vi "Initialize_Flatten.vi"(8 "error in":errorcluster, 10 "InstanceName":string, 11 "ChillerNew.lvclass":refnum<class "ChillerNew.lvclass">) -> (0 "error out":errorcluster, 3 "output cluster":refnum<class "ChillerNew.lvclass">)   [LabVIEW 2023, in "ChillerNew.lvclass"]
uses:
  ChillerNew.lvclass
  ChillerNew.lvclass/ChillerNew.ctl
  287c8f4c-a7e3-4bef-a246-9f8e491f331f.vi
  026c2e1f-36c0-42b1-b36e-75aff64539ee.vi
  f03e60db-0e78-4351-a110-c32dc1ba0a1a.vi
  838db0e1-c7d3-41be-87a2-4c748dcee471.vi
  026c2e1f-36c0-42b1-b36e-75aff64539ee.vi/4bc1c15b-36ab-481f-b8dd-c64075ce723a.vi
  838db0e1-c7d3-41be-87a2-4c748dcee471.vi/4bc1c15b-36ab-481f-b8dd-c64075ce723a.vi
  <vilib>/ADAS Replay HIL/AdasHilServices/AdasHilServices Fill In Error Info Ex.vi
  <vilib>/Utility/Data Type/NI_Data Type.lvlib
  AdasHilServices.dll
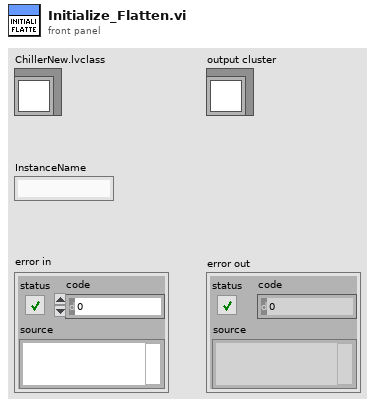
[diagram p1: front panel]
types:
  T1 = cluster{"OnOffCtl":bool, "SP1":dbl, "Watchdog":i32}
  T2 = cluster{"OnOffSts":bool, "AV1":dbl, "WatchdogSTS":i32}
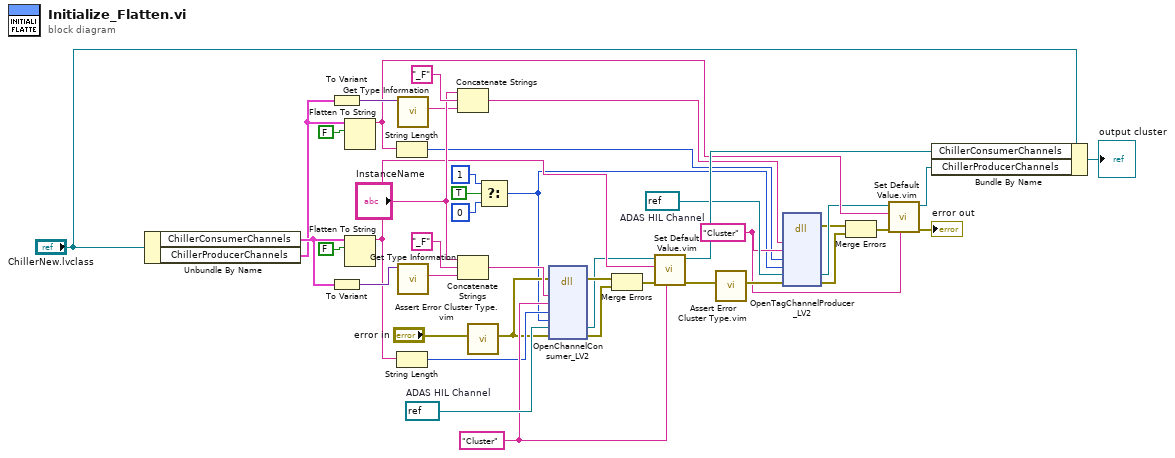
[diagram p0: block diagram]
diagram:
  w8 = refnum<k21> refnum  # ADAS HIL Channel
  w26 = refnum<k21> refnum  # ADAS HIL Channel
  w20 = "Cluster" ("Channel Type Description")
  w4 = "Cluster" ("Channel Type Description")
  n1 = Unbundle By Name("ChillerNew.lvclass") -> ("ChillerConsumerChannels"=w29:T1, "ChillerProducerChannels"=w27:T2)
  n2 = To Variant(anything=w27) -> (Variant=w41:variant)
  n3 = To Variant(anything=w29) -> (Variant=w42:variant)
  n4 = Flatten To String(anything=w27, prepend array or string size? (T)=FALSE) -> (data string=w14:string)  [unwired: 2 in, 2 out]
  n5 = Flatten To String(anything=w29, prepend array or string size? (T)=FALSE) -> (data string=w19:string)  [unwired: 2 in, 2 out]
  n6 = String Length(string=w14) -> (length=w3:i32)
  n7 = String Length(string=w19) -> (length=w18:i32)
  n8 = call <vilib>:"Get Type Information.vi"("variant"=w41) -> ("name"=w36:string)  [unwired: 6 in, 4 out]
  n9 = call <vilib>:"Get Type Information.vi"("variant"=w42) -> ("name"=w39:string)  [unwired: 6 in, 4 out]
  n10 = Concatenate Strings("InstanceName", "_F" ("string"), w36) -> (w5:string)
  n11 = Concatenate Strings("InstanceName", "_F" ("string"), w39) -> (w21:string)
  n12 = call "Assert Error Cluster Type.vim"("value in"="error in") -> ("value out"=w12:errorcluster)  [unwired: 8 in]
  n13 = Select(t=u32 1, s=TRUE ("Create if not found? (T)"), f=u32 0 ("t")) -> (s? t:f=w2:u32)
  n14 = dll-call lib="AdasHilServices.*" fn="OpenChannelConsumer_LV2"(error in=w12, "channelName"=w21, "channelTypeDescription"=w20, "elementSize"=w18, "flags"=w2, "handleOut"=w26, "error"=w12) -> (error out=w25:errorcluster, "handleOut"=w15:refnum<k21>, "error"=w24:errorcluster)  [unwired: 7 in, 1 out]
  n15 = Merge Errors(w25, w24) -> (w10:errorcluster)
  n16 = call "Set Default Value.vim"("Channel Type Description"=w20, "error in"=w10, "Data in"=w19, "ADAS HIL Channel in"=w15) -> ("error out"=w13:errorcluster, "ADAS HIL Channel out"=w31:refnum<k21>)  [unwired: 6 in]
  n17 = call "Assert Error Cluster Type.vim"("value in"=w13) -> ("value out"=w9:errorcluster)  [unwired: 8 in]
  n18 = dll-call lib="AdasHilServices.*" fn="OpenTagChannelProducer_LV2"("channelName"=w5, "channelTypeDescription"=w4, "elementSize"=w3, "flags"=w2, "handleOut"=w8, "error"=w9) -> (error out=w1:errorcluster, "handleOut"=w7:refnum<k21>, "error"=w6:errorcluster)  [unwired: 8 in, 1 out]
  n19 = Merge Errors(w1, w6) -> (w11:errorcluster)
  n20 = call "Set Default Value.vim"("Channel Type Description"=w4, "error in"=w11, "Data in"=w14, "ADAS HIL Channel in"=w7) -> ("error out"=→"error out":errorcluster, "ADAS HIL Channel out"=w32:refnum<k21>)  [unwired: 6 in]
  n21 = Bundle By Name(cluster="ChillerNew.lvclass", "ChillerConsumerChannels"=w31, "ChillerProducerChannels"=w32) -> (→"output cluster":refnum<class "ChillerNew.lvclass">)
